vi "Create.vi"(8 "error in (no error)":errorcluster) -> (0 "error out":errorcluster, 3 "Controller out":refnum<class "Controller.lvclass">)   [LabVIEW 2020, in "UIContainer.lvlib" / "Controller.lvclass"]
uses:
  Controller.lvclass
  View/View.lvclass
  C:/Users/N Tan/Documents/2-Prototypes/MVC/UIContainer/iView/iView.lvclass
  Controller.lvclass/Controller.ctl
  UIHome/Controller/Controller.lvclass
  C:/Users/N Tan/Documents/2-Prototypes/MVC/UIContainer/View/View.lvclass
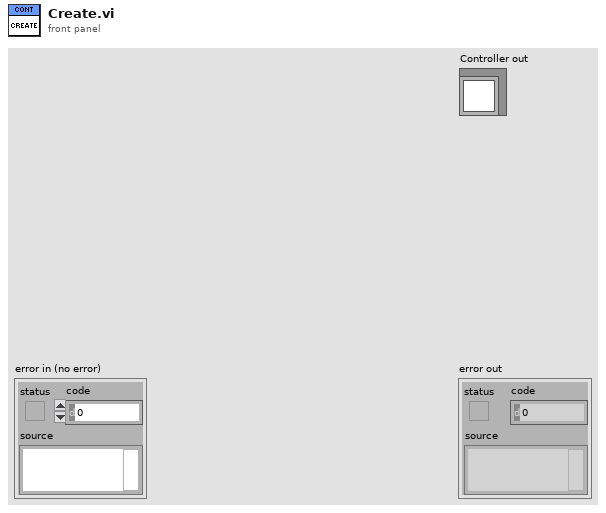
[diagram p1: front panel]
types:
  T1 = cluster{"Controller out":refnum<class "Controller.lvclass">}
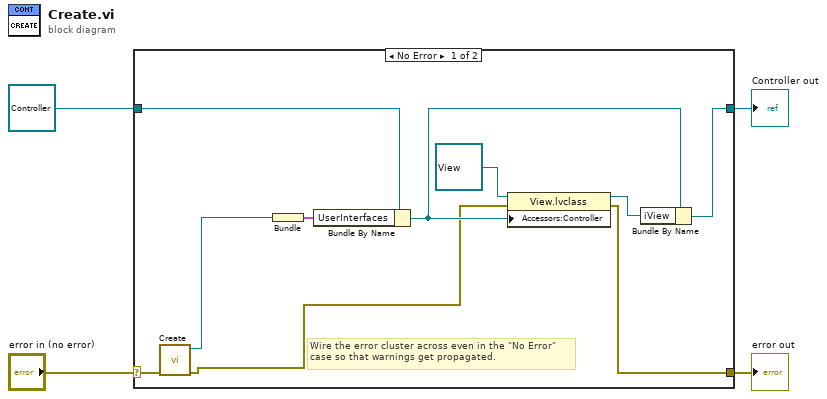
[diagram p0: block diagram]
diagram:
  n1 = case shown="No Error" "error in (no error)" {
    selector: "error in (no error)" -> [w7 w16]
    tunnel: [w9 w16] -> w3
    tunnel: [w10 w15] -> w2
    tunnel: refnum<class "Controller.lvclass"> refnum ("Controller in") -> [w14 w15]
    frame No Error {
      # "Wire the error cluster across even in the \"No Error\"\ncase so that warnings get propagated."
      n2 = call "Create.vi"("error in (no error)"=w7) -> ("error out"=w5:errorcluster, "Controller out"=w8:refnum<class "Controller.lvclass">)  [unwired: 9 in]
      n3 = Bundle("Controller out"=w8) -> (w6:T1)  [unwired: 1 in]
      n4 = Bundle By Name(cluster=w14, "UserInterfaces"=w6) -> (w11:refnum<class "Controller.lvclass">)
      n5 = property class="View.lvclass"(reference=refnum<class "View.lvclass"> refnum ("UIContainer.lvlib:View.lvclass"), error in=w5, "Accessors:Controller"=w11) -> (reference out=w12:refnum<class "View.lvclass">, error out=w9:errorcluster)
      n6 = Bundle By Name(cluster=w11, "iView"=w12) -> (w10:refnum<class "Controller.lvclass">)
    }
    frame Error {
    }
  }
  "error out" <- w3
  "Controller out" <- w2
